vi "General I2C Write Example.vi"() -> ()   [LabVIEW 2014]
doc: "This EEPROM example shows a more generalized way to use the I2C basic API to write data. It allows the user to change the following parameters: page size, write delay, the endianness of the address bytes, and the number of bytes in an address.\n\nThe parameters will have the following effects:\n\nTarget Page Size (bytes): This places an additional constraint on the amount of bytes written. The smaller value will be used, and that number of bytes written.\nWrite Delay Between Pages (ms): This will force a mandatory delay after writing bytes to a device.\nData Address Width: This will allow the user to specify the EEPROM Data Address as either 1 or 2 bytes.\nData Address Endianness: This control will change the ordering of the bytes in the EEPROM Data Address, note that this only has an effect if there are 2 bytes in the address.\n\nSince the I2C SDA and SCL lines are open-drain, they must be pulled up to the required reference voltage of your slave by connecting an appropriate resistor (2k-5k) between SCL and your reference voltage and SDA and your reference voltage. For NI-845x Hardware that contain internal pull-ups, you can use these. Otherwise, you need to use external pullups.\n\nFor connection information see the NI-845x Hardware and Software manual and the manual for your specific EEPROM."
uses:
  <vilib>/ni845x/ni845x.llb/ni845xControl.ctl
  <vilib>/ni845x/ni845x.llb/NI-845x I2C Close Configuration Reference.vi
  <resource>/objmgr/NI845x.rc
panel:
  in  "I/O Voltage Level":i32(ring)=33 items=["3.3V"=33, "2.5V"=25, "1.8V"=18, "1.5V"=15, "1.2V"=12]
  in  "Use Internal I2C Pullup Resistor":bool
  in  "Data Address Width":enum16{"1 Byte", "2 Byte"}(ring)=enum."2 Byte"
  in  "Data Address Endianness":bool=TRUE
  in  "Write Delay Between Pages (ms)":u32=4
  in  "Target Page Size (bytes)":u32=128
  in  "EEPROM Data Address":u16 format="%.0x"
  in  "Number of Bytes to Write":u32=128
  in  "Clock Rate (kHz)":u16=100
  in  "Address":u16=80 format="%.0x"
  out "Data Bytes Written":u8[](array[numeric]) format="%x"
  in  "Device":T1
  # "See VI Info <Ctrl+I> for more information on how to use this example"
  # "Device Configuration"
  # "I2C Data"
  # "I2C Slave Configuration"
  # "Big Endian"
  # "Little Endian"
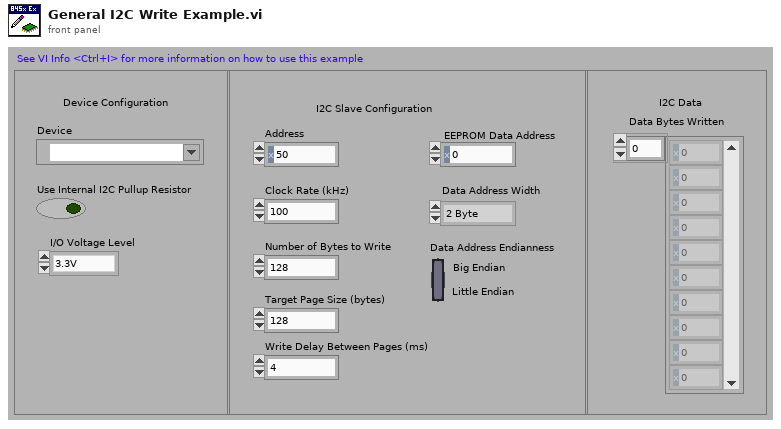
[diagram p1: front panel]
types:
  T1 = typedef "ni845xControl.ctl" = refnum<k21>
  T2 = typedef "ni845xI2cConfiguration.ctl" = refnum<k20>
  T3 = cluster{"EEPROM Address":u16, "Length":u32, "Data Index":u32}[]
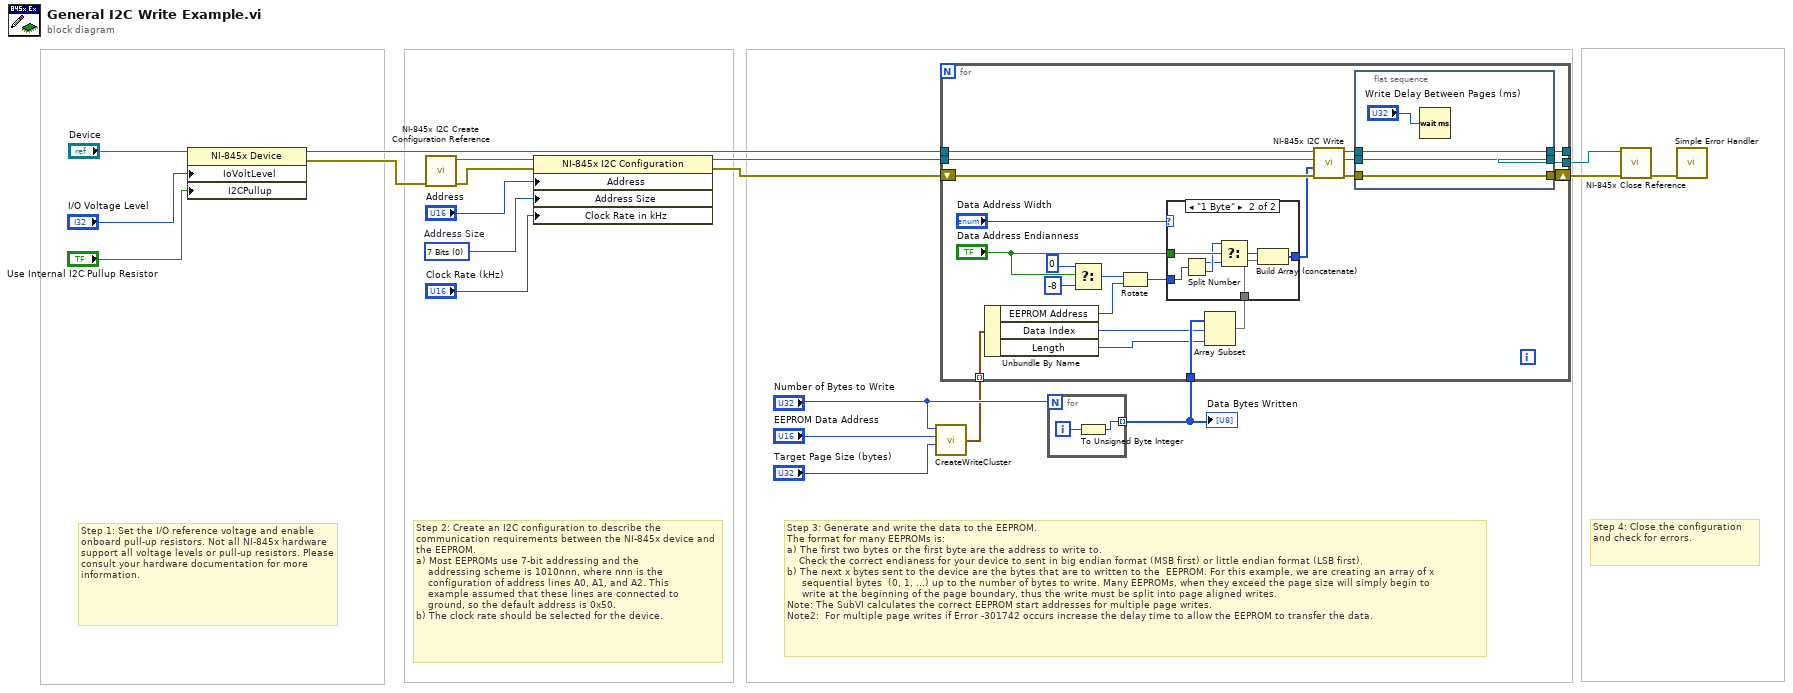
[diagram p0: block diagram]
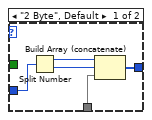
[diagram p2: hidden frame]
diagram:
  w19 = 0 items=["7 Bits", "10 Bits"]  # Address Size
  # "Step 1: Set the I/O reference voltage and enable onboard pull-up resistors. Not all NI-845x hardware support all voltage levels or pull-up resistors. Please consult your hardware documentation for more information."
  # "Step 4: Close the configuration \nand check for errors."
  # "Step 2: Create an I2C configuration to describe the \ncommunication requirements between the NI-845x device and the EEPROM.\na) Most EEPROMs use 7-bit addressing and the\n    addressing scheme is 1010nnn, where nnn is the\n    configuration of address lines A0, A1, and A2. This    \n    example assumed that these lines are connected to\n    ground, so the default address is 0x50. \nb) The clock rate should be selected for the device."
  # "Step 3: Generate and write the data to the EEPROM. \nThe format for many EEPROMs is:\na) The first two bytes or the first byte are the address to write to. \n    Check the correct endianess for your device to sent in big endian format (MSB first) or little endian format (LSB first).\nb) The next x bytes sent to the device are the bytes that are to written to the  EEPROM. For this example, we are creating an array of x\n     sequential bytes  (0, 1, ...) up to the number of bytes to write. Many EEPROMs, when they exceed the page size will simply begin to\n     write at the beginning of the page boundary, thus the write must be split into page aligned writes.\nNote: The SubVI calculates the correct EEPROM start addresses for multiple page writes.\nNote2:  For multiple page writes if Error -301742 occurs increase the delay time to allow the EEPROM to transfer the data."
  n1 = property on="Property Node" class="NI-845x Device"(reference="Device", "IoVoltLevel"="I/O Voltage Level", "I2CPullup"="Use Internal I2C Pullup Resistor") -> (reference out=w4:T1, error out=w3:errorcluster)  [unwired: 1 in]
  n2 = call <vilib>:"NI-845x I2C Create Configuration Reference.vi"("error in (no error)"=w3) -> ("error out"=w15:errorcluster, "i2c configuration"=w16:T2)  [unwired: 9 out]
  n3 = property on="Property Node" class="NI-845x I2C Configuration"(reference=w16, error in=w15, "Address"="Address", "Address Size"=w19, "Clock Rate in kHz"="Clock Rate (kHz)") -> (reference out=w13:T2, error out=w12:errorcluster)
  n4 = call "CreateWriteCluster.vi"("Page Size in Bytes"="Target Page Size (bytes)", "EEPROM Starting Address"="EEPROM Data Address", "Number of Bytes to Write"="Number of Bytes to Write") -> ("Array of Write Cluster Information"=w6:T3)  [unwired: 1 out]
  n5 = for {
    N: "Number of Bytes to Write" -> [_]
    tunnel: [w22] -> w9 mode=indexing
    i -> [w21]
    n6 = To Unsigned Byte Integer(number=w21) -> (unsigned 8bit integer=w22:u8)
  }
  "Data Bytes Written" <- w9
  n7 = for {
    shift-right: [w44] -> w14
    shift-left: w12 -> [w41]
    tunnel: w9 -> [w28]
    tunnel: w4 -> [w39]
    tunnel: [w43] -> _
    tunnel: w13 -> [w42]
    tunnel: [w31] -> w11
    tunnel: w6 -> [w24] mode=indexing
    n8 = Unbundle By Name(w24) -> ("EEPROM Address"=w25:u16, "Data Index"=w26:u32, "Length"=w27:u32)
    n9 = Select(t=i16 0, s="Data Address Endianness", f=i16 -8) -> (s? t:f=w35:i16)
    n10 = Rotate(1:w25, 2:w35) -> (0:w34:u16)
    n11 = Array Subset(array=w28, index=w26, length=w27) -> (w30:u8[])
    n12 = case shown="\"1 Byte\"" "Data Address Width" {
      tunnel: w34 -> [w49 w54]
      tunnel: [w48 w56] -> w23
      tunnel: w30 -> [w47 w55]
      tunnel: "Data Address Endianness" -> [_ w53]
      frame "2 Byte", Default {
        n13 = Split Number(x=w49) -> (hi(x)=w45:u8, lo(x)=w46:u8)
        n14 = Build Array (concatenate)(w45, w46, w47) -> (w48:u8[])
      }
      frame "1 Byte" {
        n15 = Split Number(x=w54) -> (hi(x)=w50:u8, lo(x)=w51:u8)
        n16 = Select(t=w51, s=w53, f=w50) -> (s? t:f=w52:u8)
        n17 = Build Array (concatenate)(w52, w55) -> (w56:u8[])
      }
    }
    n18 = call <vilib>:"NI-845x I2C Write.vi"("error in (no error)"=w41, "write data"=w23, "i2c configuration in"=w42, "device reference in"=w39) -> ("error out"=w40:errorcluster, "i2c configuration out"=w32:T2, "device reference out"=w38:T1)  [unwired: 5 out]
    n19 = flat-sequence {
      tunnel: [w60] -> w44
      tunnel: [w59] -> w43
      tunnel: w38 -> [w59]
      tunnel: w40 -> [w60]
      tunnel: w32 -> [w58]
      tunnel: [w58] -> w31
      frame #0 {
        n20 = Wait (ms)(milliseconds to wait="Write Delay Between Pages (ms)") -> ()  [unwired: 1 out]
      }
    }
  }
  n21 = call-poly <vilib>:"NI-845x Close Reference.vi"("error in (no error)"=w14, "i2c configuration"=w11) -> ("error out"=w17:errorcluster)  [unwired: 9 out]
  n22 = call <vilib>:"Simple Error Handler.vi"("error in (no error)"=w17) -> ()  [unwired: 1 in, 8 out]
